vi "Test X-Stage.vi"() -> ()   [LabVIEW 2014]
uses:
  Controls/Translation Stage Cluster.ctl
  General/Controls/Translation Stage Types.ctl
  General/Controls/Set Get Controls.ctl
  Controls/Motion Translation Module Control.ctl
panel:
  out "Cluster Out":T1={"Position"=0.0, "Is.Enabled?"=FALSE, "Is.Connected?"=FALSE, "Device SN"="45876539", "AccelerationMaximum"=0.0, "VelocityMaximum"=0.0, "Acceleration"=0.0, "Velocity"=0.0, "waitTimeout (ms)"=0, "Model"=enum."None", "Is.Homed?"=FALSE}
  out "Error Out":errorcluster
  in  "Uninit":bool
  in  "Cluster In":T1={"Position"=0.0, "Is.Enabled?"=FALSE, "Is.Connected?"=FALSE, "Device SN"="45876539", "AccelerationMaximum"=0.0, "VelocityMaximum"=0.0, "Acceleration"=0.0, "Velocity"=0.0, "waitTimeout (ms)"=0, "Model"=enum."None", "Is.Homed?"=FALSE}
  in  "Init":bool
  in  "Cancel Button":bool
  in  "Position":bool
  in  "Stop":bool
  in  "Home":bool
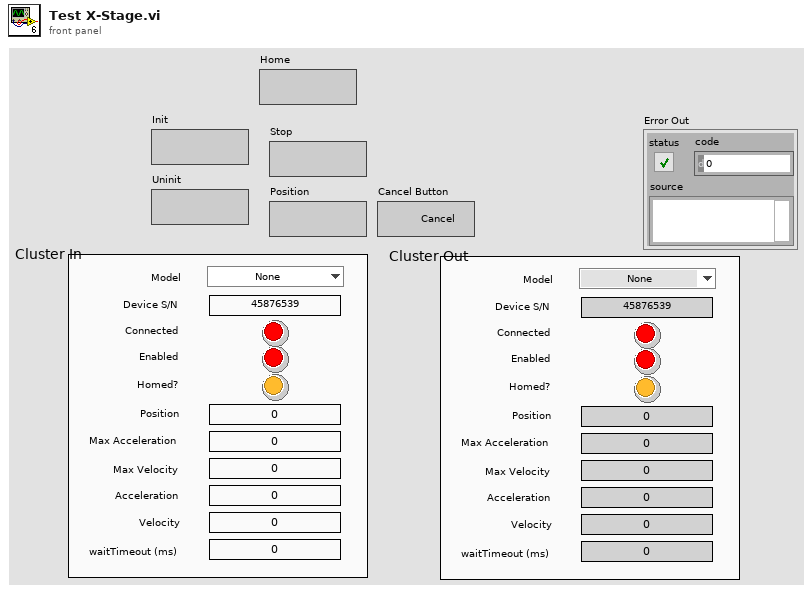
[diagram p1: front panel]
types:
  T1 = typedef "Translation Stage Cluster.ctl" = cluster{"Position":dbl, "Is.Enabled?":bool, "Is.Connected?":bool, "Device SN":string, "AccelerationMaximum":dbl, "VelocityMaximum":dbl, "Acceleration":dbl, "Velocity":dbl, "waitTimeout (ms)":i32, "Model":T2, "Is.Homed?":bool}
  T2 = typedef "Translation Stage Types.ctl" = enum16{"None", "Thorlabs LTS", "Thorlabs MLJ"}
  T3 = typedef "Motion Translation Module Control.ctl" = enum16{"Init", "Home", "Configure", "Velocity/Accel", "Position", "Jog", "Stop", "Uninit"}
  T4 = typedef "Set Get Controls.ctl" = enum16{"Set", "Get"}
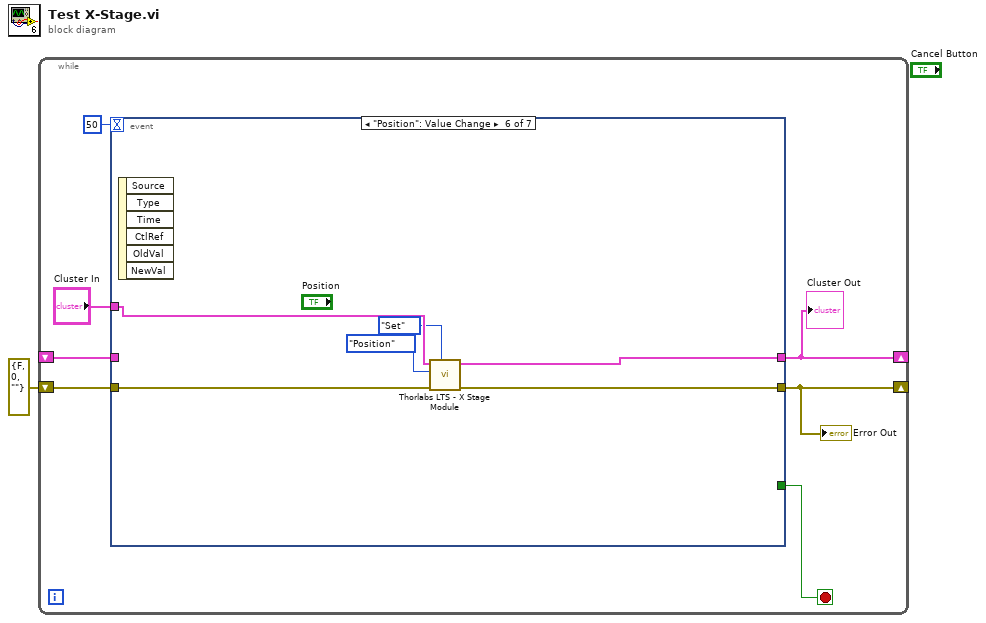
[diagram p0: block diagram]
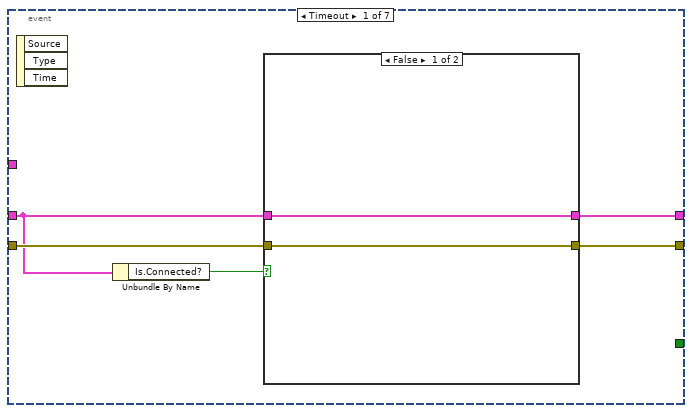
[diagram p2: hidden frame]
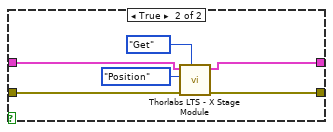
[diagram p3: hidden frame]
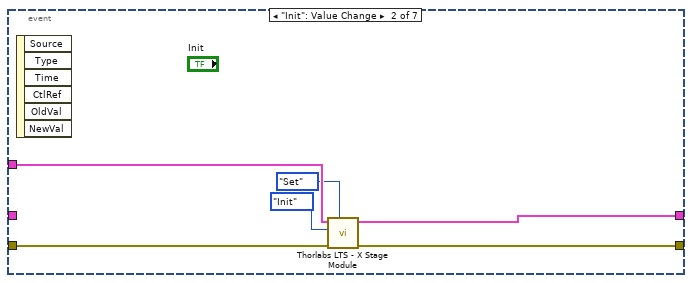
[diagram p4: hidden frame]
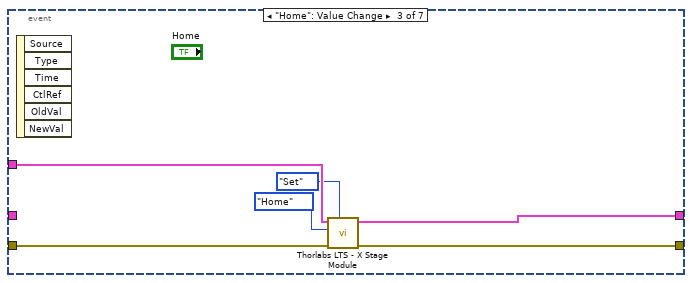
[diagram p5: hidden frame]
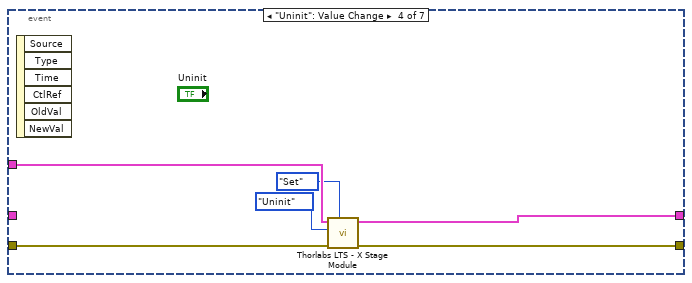
[diagram p6: hidden frame]
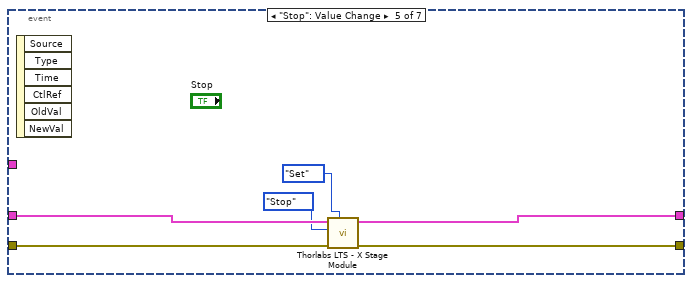
[diagram p7: hidden frame]
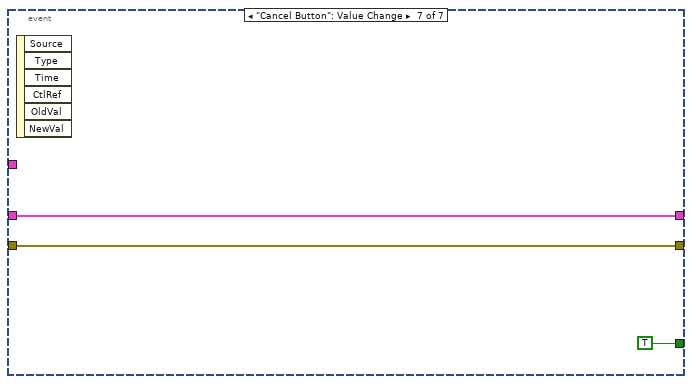
[diagram p8: hidden frame]
diagram:
  n1 = while {
    shift-right: [w6] -> _
    shift-left: errorcluster {"status"=FALSE, "code"=0, "source"=""} ("Error Out") -> [w5]
    shift-right: [w3] -> _
    shift-left: _ -> [w4]
    stop <- w7 stop-if-true
    n2 = event shown="[5] \"Position\": Value Change" {
      selector: _ -> [_ _ _ _ _ _ _]
      dyn-events: _ -> [_ _ _ _ _ _ _]
      timeout: 50 -> [_ _ _ _ _ _ _]
      tunnel: [_ _ _ _ _ _ TRUE] -> w7
      tunnel: [w13 w25 w31 w37 w43 w49 w53] -> w3
      tunnel: w4 -> [w10 _ _ _ w42 _ w53]
      tunnel: [w12 w26 w32 w38 w44 w50 w52] -> w6
      tunnel: w5 -> [w11 w27 w33 w39 w45 w51 w52]
      tunnel: "Cluster In" -> [_ w23 w29 w35 _ w47 _]
      event Timeout {
        n3 = event-data() -> ()  [unwired: 1 in, 3 out]
        n4 = Unbundle By Name(w10) -> ("Is.Connected?"=w9:bool)
        n5 = case shown="False" w9 {
          tunnel: [w15 w19] -> w13
          tunnel: [w14 w18] -> w12
          tunnel: w11 -> [w14 w17]
          tunnel: w10 -> [w15 w16]
          frame False {
          }
          frame True {
            n6 = call "Thorlabs LTS - X Stage Module.vi"("Set/Get"=Set_Get_Controls."Get", "Error In"=w17, "Action"=Motion_Translation_Module_Control."Position", "Cluster In"=w16) -> ("Error Out"=w18:errorcluster, "Cluster Out"=w19:T1)  [unwired: 6 in]
          }
        }
      }
      event "Init": Value Change {
        n7 = event-data() -> ()  [unwired: 1 in, 6 out]
        n8 = call "Thorlabs LTS - X Stage Module.vi"("Set/Get"=Set_Get_Controls."Set", "Error In"=w27, "Action"=Motion_Translation_Module_Control."Init", "Cluster In"=w23) -> ("Error Out"=w26:errorcluster, "Cluster Out"=w25:T1)  [unwired: 6 in]
      }
      event "Home": Value Change {
        n9 = event-data() -> ()  [unwired: 1 in, 6 out]
        n10 = call "Thorlabs LTS - X Stage Module.vi"("Set/Get"=Set_Get_Controls."Set", "Error In"=w33, "Action"=Motion_Translation_Module_Control."Home", "Cluster In"=w29) -> ("Error Out"=w32:errorcluster, "Cluster Out"=w31:T1)  [unwired: 6 in]
      }
      event "Uninit": Value Change {
        n11 = event-data() -> ()  [unwired: 1 in, 6 out]
        n12 = call "Thorlabs LTS - X Stage Module.vi"("Set/Get"=Set_Get_Controls."Set", "Error In"=w39, "Action"=Motion_Translation_Module_Control."Uninit", "Cluster In"=w35) -> ("Error Out"=w38:errorcluster, "Cluster Out"=w37:T1)  [unwired: 6 in]
      }
      event "Stop": Value Change {
        n13 = event-data() -> ()  [unwired: 1 in, 6 out]
        n14 = call "Thorlabs LTS - X Stage Module.vi"("Set/Get"=Set_Get_Controls."Set", "Error In"=w45, "Action"=Motion_Translation_Module_Control."Stop", "Cluster In"=w42) -> ("Error Out"=w44:errorcluster, "Cluster Out"=w43:T1)  [unwired: 6 in]
      }
      event "Position": Value Change {
        n15 = event-data() -> ()  [unwired: 1 in, 6 out]
        n16 = call "Thorlabs LTS - X Stage Module.vi"("Set/Get"=Set_Get_Controls."Set", "Error In"=w51, "Action"=Motion_Translation_Module_Control."Position", "Cluster In"=w47) -> ("Error Out"=w50:errorcluster, "Cluster Out"=w49:T1)  [unwired: 6 in]
      }
      event "Cancel Button": Value Change {
        n17 = event-data() -> ()  [unwired: 1 in, 6 out]
      }
    }
    "Error Out" <- w6
    "Cluster Out" <- w3
  }
